vi "JA_Get.vi"(8 "error in (no error)":errorcluster, 10 "Axis Number":i32, 11 "Agilis in":T2) -> (0 "error out":errorcluster, 2 "Jog Mode":T1 items=["-666 steps/s"=-4, "-1700 steps/s"=-3, "-100 steps/s"=-2, "-5 steps/s"=-1, "No move"=0, "+5 steps/s"=1, "+100 steps/s"=2, "+1700 steps/s"=3, "+666 steps/s"=4], 3 "Agilis out":T2)   [LabVIEW 2016, in "Drivers.lvlib" / "Agilis.lvlib"]
doc: "Returns current jog mode."
uses:
  Agilis.lvlib
  AgilisCmdLib Refnum.ctl
  Jog Mode.ctl
  Z:/TraceGrabber/Drivers/Agilis/AgilisCmdLib.dll
  AgilisCmdLib.dll
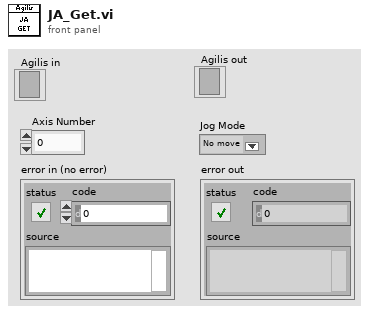
[diagram p1: front panel]
types:
  T1 = typedef "Drivers.lvlib/Agilis.lvlib/Jog Mode.ctl" = i32
  T2 = typedef "Drivers.lvlib/Agilis.lvlib/AgilisCmdLib Refnum.ctl" = refnum<k24>
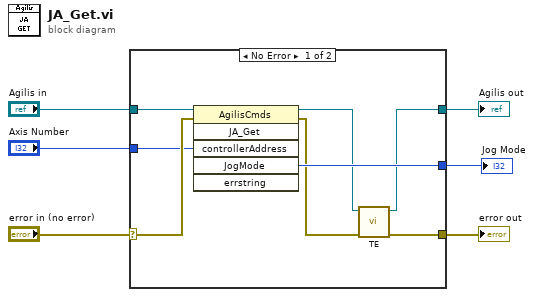
[diagram p0: block diagram]
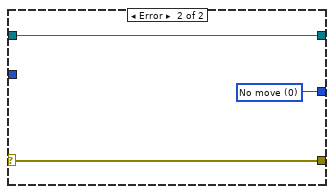
[diagram p2: hidden frame]
diagram:
  n1 = case shown="No Error" "error in (no error)" {
    selector: "error in (no error)" -> [w13 w17]
    tunnel: "Agilis in" -> [w14 w16]
    tunnel: [w7 w16] -> w4
    tunnel: [w10 w17] -> w3
    tunnel: "Axis Number" -> [w12 _]
    tunnel: [w11 w15] -> w1
    frame No Error {
      n2 = invoke class="AgilisCmds" method="JA_Get"(reference=w14, error in=w13, "controllerAddress"=w12) -> (reference out=w8:T2, error out=w9:errorcluster, "JogMode"=w11:i32)  [unwired: 3 in, 3 out]
      n3 = call "TE.vi"("error in (no error)"=w9, "Agilis in"=w8) -> ("error out"=w10:errorcluster, "Agilis out"=w7:T2)  [unwired: 8 in]
    }
    frame Error {
      w15 = T1 0 items=["-666 steps/s"=-4, "-1700 steps/s"=-3, "-100 steps/s"=-2, "-5 steps/s"=-1, "No move"=0, "+5 steps/s"=1, "+100 steps/s"=2, "+1700 steps/s"=3, "+666 steps/s"=4] ("Jog Mode 2")
    }
  }
  "Agilis out" <- w4
  "error out" <- w3
  "Jog Mode" <- w1
